vi "DestroyEvents.vi"(8 "error in (no error)":errorcluster, 11 "Events":T1) -> (0 "error out":errorcluster)   [LabVIEW 2020, in "Signal Generation.lvlib"]
uses:
  Signal Generation.lvlib
  Controls/SignalParamTD.ctl
  Controls/SignalShapeTD.ctl
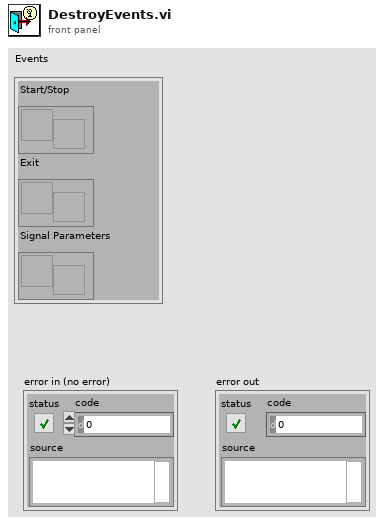
[diagram p1: front panel]
types:
  T1 = cluster{"Start/Stop":refnum<user-event>, "Exit":refnum<user-event>, "Signal Parameters":refnum<user-event>}
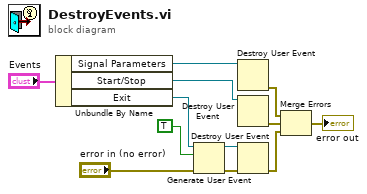
[diagram p0: block diagram]
diagram:
  n1 = Unbundle By Name("Events") -> ("Signal Parameters"=w2:refnum<user-event>, "Start/Stop"=w12:refnum<user-event>, "Exit"=w11:refnum<user-event>)
  n2 = Generate User Event(user event=w11, event data cluster=TRUE ("event data"), error in="error in (no error)") -> (user event out=w10:refnum<user-event>, error out=w8:errorcluster)  [unwired: 1 in]
  n3 = Destroy User Event(user event=w2) -> (error out=w1:errorcluster)  [unwired: 1 in]
  n4 = Destroy User Event(user event=w12) -> (error out=w6:errorcluster)  [unwired: 1 in]
  n5 = Destroy User Event(user event=w10, error in=w8) -> (error out=w7:errorcluster)
  n6 = Merge Errors(w1, w6, w7) -> (→"error out":errorcluster)
